vi "ifr2025 Modulation  .vi"(0 "instrument handle":refnum<visa-resource-name>, 7 "Channel (AM1)":i16(ring)=1 items=["AM", "AM1", "AM2", "FM", "FM1", "FM2", "PM", "PM1", "PM2"], 11 "error in (no error)":errorcluster {"code" format="%.0x"}) -> (2 "State":i16, 3 "Source":i16, 4 "instrument handle out":refnum<visa-resource-name>, 6 "Depth/Deviation":dbl, 8 "Depth/Dev Increment":dbl, 10 "Frequency":dbl, 13 "Shape":i16, 14 "Frequency Increment":dbl, 15 "error out":errorcluster {"code" format="%.0x"})   [LabVIEW 2009]
doc: "Returns information about any of the modulation sources."
uses:
  Ifr2025_32.dll
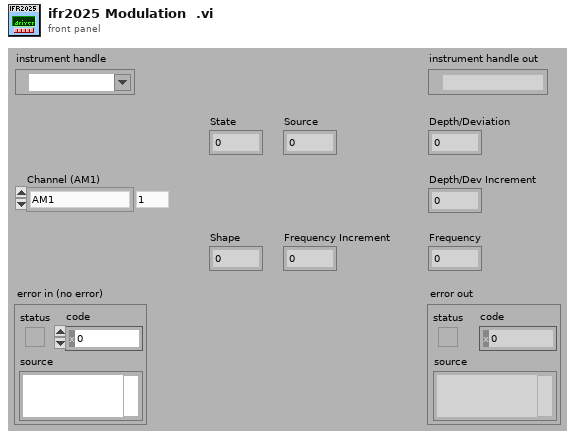
[diagram p1: front panel]
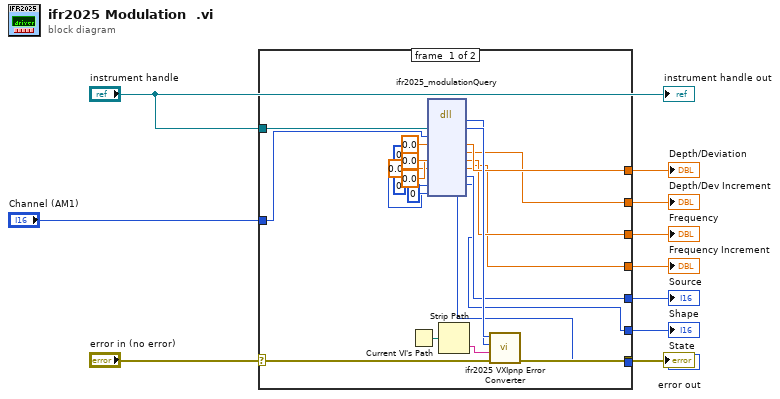
[diagram p0: block diagram]
diagram:
  n1 = case shown="No Error" "error in (no error)" {
    selector: "error in (no error)" -> [w28 w34]
    tunnel: [w27 w34] -> w11
    tunnel: "instrument handle" -> [w32 _]
    tunnel: "Channel (AM1)" -> [w26 _]
    tunnel: [w24 _] -> w7
    tunnel: [w22 _] -> w6
    tunnel: [w20 _] -> w5
    tunnel: [w18 _] -> w4
    tunnel: [w16 _] -> w3
    tunnel: [w14 _] -> w2
    tunnel: [w12 _] -> w1
    frame #0 {
      n2 = Current VI's Path() -> (path=w33:path)
      n3 = dll-call lib="P:/inst/Marconi 2024 Signal Generator/source/labview/ifr2025/ifr2025/ifr2025_*.*" fn="ifr2025_modulationQuery"("vi"=w32, "Channel"=w26, "Depth/Deviation"=0.0, "Depth/Dev Increment"=0.0, "Frequency"=0.0, "Frequency Increment"=0.0, "Source"=i16 0, "Shape"=i16 0, "State"=i16 0) -> (w30:i32, "vi"=w31:u32, "Depth/Deviation"=w24:dbl, "Depth/Dev Increment"=w22:dbl, "Frequency"=w20:dbl, "Frequency Increment"=w18:dbl, "Source"=w16:i16, "Shape"=w14:i16, "State"=w12:i16)  [unwired: 4 in, 2 out]
      n4 = Strip Path(path=w33) -> (name=w29:string)  [unwired: 1 out]
      n5 = call "ifr2025 VXIpnp Error Converter.vi"("error in (no error)"=w28, "name of VI (\"\")"=w29, "CVI error code (0)"=w30, "instrument handle"=w31) -> ("error out"=w27:errorcluster)  [unwired: 7 out]
    }
    frame #1 {
    }
  }
  "error out" <- w11
  "Depth/Deviation" <- w7
  "Depth/Dev Increment" <- w6
  "Frequency" <- w5
  "Frequency Increment" <- w4
  "Source" <- w3
  "Shape" <- w2
  "State" <- w1
  "instrument handle out" <- "instrument handle"
